vi "Do.vi"(8 "error in (no error)":errorcluster, 10 "Actor in":refnum<class "Actor.lvclass">, 11 "Ping Msg":refnum<class "Ping Msg.lvclass">) -> (0 "error out":errorcluster, 2 "Actor out":refnum<class "Actor.lvclass">)   [LabVIEW 2017, in "AF Debug.lvlib" / "Ping Msg.lvclass"]
doc: "This VI delivers the Ping Msg to any actor. This VI does not invoke any methods on the actor. It simply returns to the sender the time delay (using the high-resolution timer) between the send and the receive of the message."
uses:
  <resource>/AFDebug/Ping msg/Ping Msg.lvclass
  <vilib>/ActorFramework/Actor/Actor.lvclass
  <resource>/AFDebug/Ping msg/Ping Msg.lvclass/Ping Msg.ctl
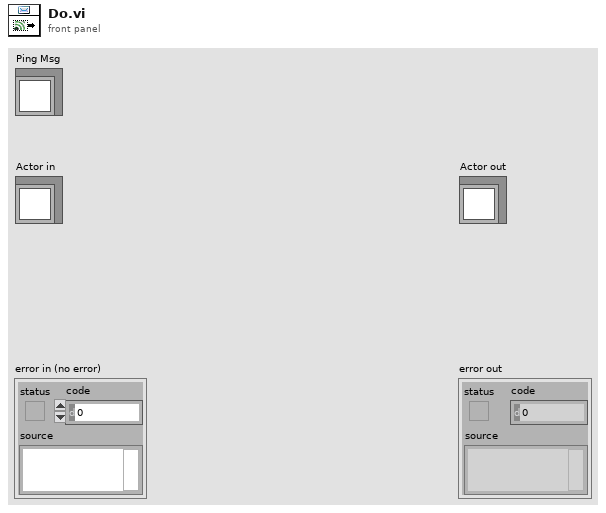
[diagram p1: front panel]
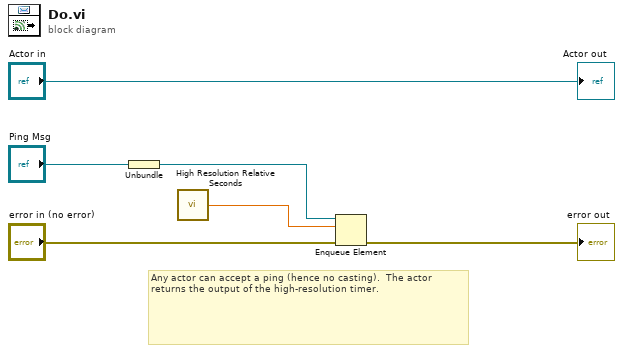
[diagram p0: block diagram]
diagram:
  # "Any actor can accept a ping (hence no casting).  The actor returns the output of the high-resolution timer."
  n1 = Unbundle("Ping Msg") -> (w2:refnum<queue>)
  n2 = call <vilib>:"High Resolution Relative Seconds.vi"() -> ("relative seconds"=w1:dbl)
  n3 = Enqueue Element(queue=w2, element=w1, error in (no error)="error in (no error)") -> (error out=→"error out":errorcluster)  [unwired: 1 in, 2 out]
  "Actor out" <- "Actor in"
